vi "Read Control Queue.vi"(8 "error in (no error)":errorcluster, 11 "Socket in":refnum<class "Execution.lvclass">) -> (0 "error out":errorcluster, 2 "Control Queue":refnum<queue>, 3 "Socket out":refnum<class "Execution.lvclass">)   [LabVIEW 2015, in "Execution.lvclass"]
uses:
  Execution.lvclass
  EXECUTION_CTRL_QUEUE_DATA.ctl
  EXECUTION_CTRL_MSG.ctl
  Execution.lvclass/Execution.ctl
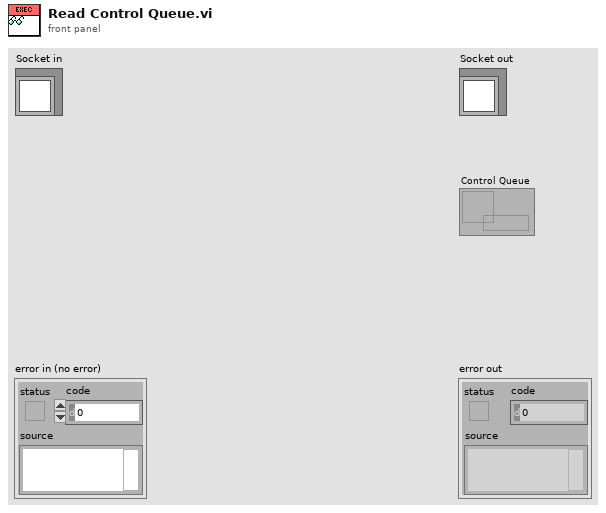
[diagram p1: front panel]
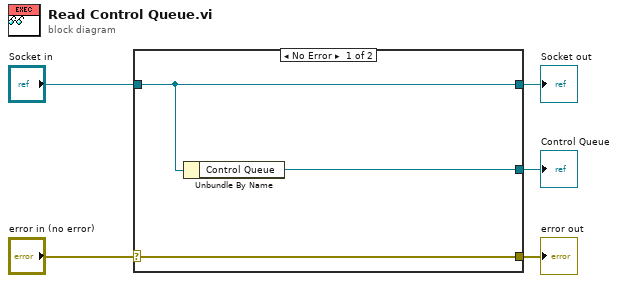
[diagram p0: block diagram]
diagram:
  n1 = case shown="No Error" "error in (no error)" {
    selector: "error in (no error)" -> [w8 w9]
    tunnel: [w8 w9] -> w4
    tunnel: [w7 w10] -> w2
    tunnel: "Socket in" -> [w7 w10]
    tunnel: [w6 _] -> w1
    frame No Error {
      n2 = Unbundle By Name(w7) -> ("Control Queue"=w6:refnum<queue>)
    }
    frame Error {
    }
  }
  "error out" <- w4
  "Socket out" <- w2
  "Control Queue" <- w1
